vi "Vision Server Ref Get.vi"(6 "Test Mode Only":bool, 8 "error in (no error)":errorcluster, 10 "refnum name":string="Vision Server RefNum") -> (0 "error out":errorcluster, 3 "VisionServerRef out":T1)   [LabVIEW 2016, in "Vision Server.lvclass"]
uses:
  Vision Server.lvclass
  typedef/Vision Server Ref.ctl
  <vilib>/Rock Robotics/WPI/Utilities/Refnum Registry Operation.ctl
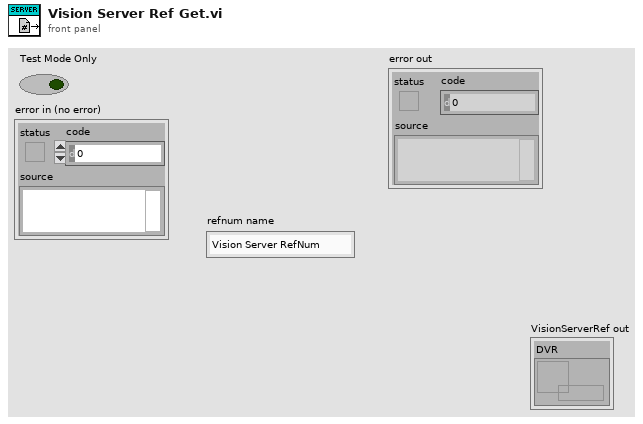
[diagram p1: front panel]
types:
  T1 = typedef "Vision Server.lvclass/Vision Server Ref.ctl" = cluster{"DVR":refnum<data-value>}
  T2 = typedef "Refnum Registry Operation.ctl" = enum16{"set", "get", "delete", "get all names", "read name"}
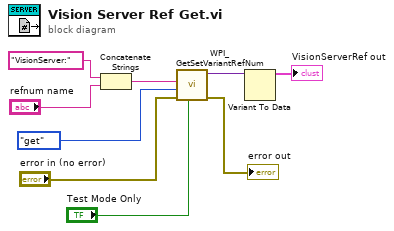
[diagram p0: block diagram]
diagram:
  n1 = Concatenate Strings("VisionServer:", "refnum name") -> (w7:string)
  n2 = call <vilib>:"WPI_GetSetVariantRefNum.vi"("Test Mode Only"="Test Mode Only", "error in (no error)"="error in (no error)", "Operation"=Refnum_Registry_Operation."get", "refnum name"=w7) -> ("error out"=→"error out":errorcluster, "DevRef"=w2:variant)  [unwired: 5 in, 1 out]
  n3 = Variant To Data(Variant=w2) -> (data=→"VisionServerRef out":T1)  [unwired: 2 in, 1 out]
